vi "FPServerQueue.vi"(11 "error in (no error)":errorcluster) -> (3 "FPServer Queue":refnum<queue>, 5 "error out":errorcluster)   [LabVIEW 2014]
uses:
  Message.ctl
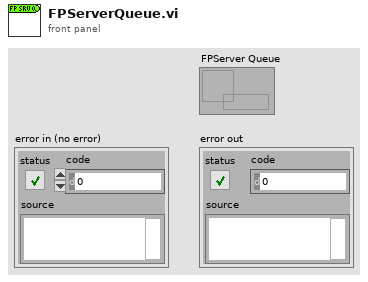
[diagram p1: front panel]
types:
  T1 = typedef "Message.ctl" = cluster{"Message":string, "Data":variant, "Response":refnum<queue>}
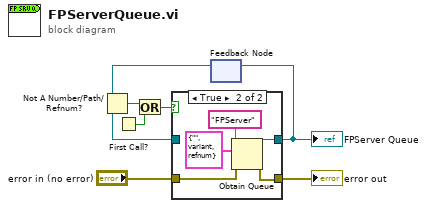
[diagram p0: block diagram]
diagram:
  n1 = First Call?() -> (First Call?: T/F=w1:bool)
  n2 = feedback #1() -> (w6:refnum<queue>)  [unwired: 1 in]
  n3 = Not A Number/Path/Refnum?(number/path/refnum=w6) -> (NaN/Path/Refnum?=w7:bool)
  n4 = Or(x=w7, y=w1) -> (x .or. y?=w2:bool)
  n5 = case shown="True" w2 {
    tunnel: [w9 w13] -> w5
    tunnel: w6 -> [w9 _]
    tunnel: "error in (no error)" -> [w8 w12]
    tunnel: [w8 w11] -> w3
    frame False {
    }
    frame True {
      n6 = Obtain Queue(name (unnamed)="FPServer", element data type=T1 {"Message"="", "Data"=variant, "Response"=refnum} ("Process Message"), error in (no error)=w12) -> (queue out=w13:refnum<queue>, error out=w11:errorcluster)  [unwired: 2 in, 1 out]
    }
  }
  "FPServer Queue" <- w5
  "error out" <- w3
  n7 = feedback-in #1(w5) -> ()
